vi "GetParam.vi"(8 "error in (no error)":errorcluster caption="entrée d'erreur (pas d'erreur)", 11 "LabelBinarizer.lvclass":refnum<class "LabelBinarizer.lvclass">) -> (0 "error out":errorcluster caption="sortie d'erreur", 2 "LabelBinarizer":T1={"neg_label"=0, "pos_label"=1, "sparse_output"=FALSE}, 3 "LabelBinarizer.lvclass":refnum<class "LabelBinarizer.lvclass">)   [LabVIEW 2020, in "LabelBinarizer.lvclass"]
doc: "Get Parameters"
uses:
  LabelBinarizer.lvclass
  LabelBinarizer.lvclass/LabelBinarizer.ctl
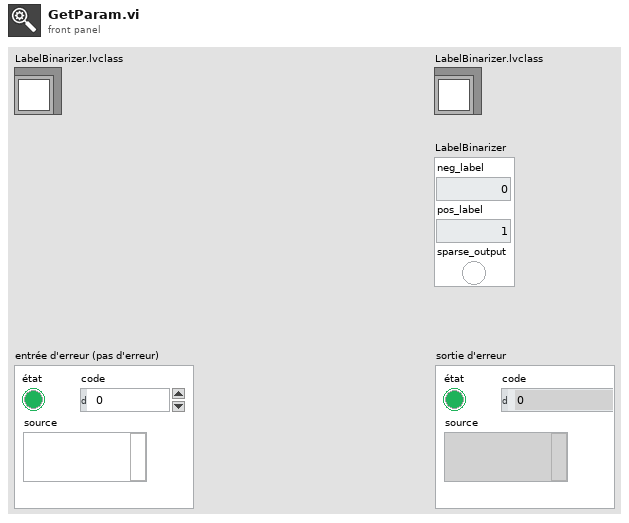
[diagram p1: front panel]
types:
  T1 = cluster{"neg_label":i32, "pos_label":i32, "sparse_output":bool}
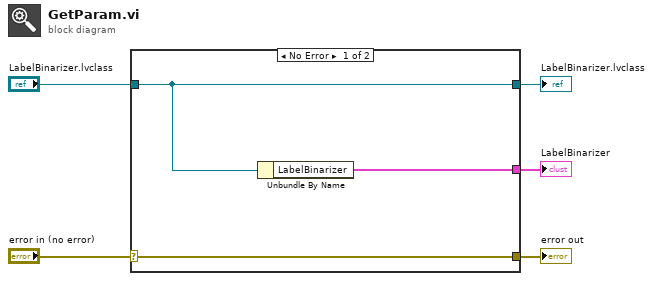
[diagram p0: block diagram]
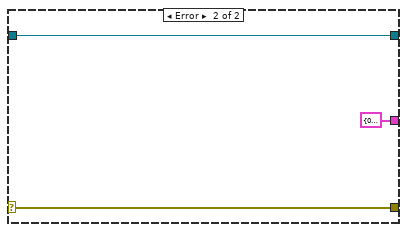
[diagram p2: hidden frame]
diagram:
  n1 = case shown="No Error" "error in (no error)" {
    selector: "error in (no error)" -> [w8 w10]
    tunnel: [w8 w10] -> w4
    tunnel: [w7 w11] -> w2
    tunnel: "LabelBinarizer.lvclass" -> [w7 w11]
    tunnel: [w6 T1 {"neg_label"=0, "pos_label"=0, "sparse_output"=FALSE} ("LabelBinarizer")] -> w1
    frame No Error {
      n2 = Unbundle By Name(w7) -> ("LabelBinarizer"=w6:T1)
    }
    frame Error {
    }
  }
  "error out" <- w4
  "LabelBinarizer.lvclass" <- w2
  "LabelBinarizer" <- w1
